vi "Test_Python_Node.vi"   [LabVIEW 2020]
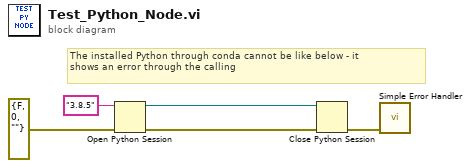
[diagram p0: block diagram]
diagram:
  # "The installed Python through conda cannot be like below - it \nshows an error through the calling"
  n1 = Open Python Session(python version="3.8.5" ("Python version"), 3:errorcluster {"status"=FALSE, "code"=0, "source"=""} ("error in (no error)")) -> (session out=w3:refnum<k35>, error out=w4:errorcluster)  [unwired: 1 in]
  n2 = Close Python Session(session in=w3, error in=w4) -> (11:w2:errorcluster)
  n3 = call <vilib>:"Simple Error Handler.vi"("error in (no error)"=w2) -> ()  [unwired: 4 in, 5 out]
